vi "挥发酚数据插入.vi"(0 "data":T1={"时间"=timestamp(0 s since 1904-01-01), "测量模式"="水样测试", "数据类型"="N", "检测值"=0.0, "单位"="mg/L", "数据标识"="N", "X0"=0.0, "标样参考值"=0.0, "跨度值"=0.0, "因子编码"="", "X^2"=0.0, "X"=0.0, "B 2"=0.0, "测量量程"=0.0, "测量检出限"=0.0, "测量精度"=0.0, "测量间隔"=0.0, "消解温度"=0.0, "消解时长"=0.0, "三项式系数"=0.0, "二次多项式系数"=0.0, "曲线斜率"=0.0, "曲线截距"=0.0, "线性相关系数"=0.0, "空白校准时间"=timestamp(0 s since 1904-01-01), "标样校准时间"=timestamp(0 s since 1904-01-01), "测量信号值"=0.0, "稀释倍数"=0.0, "量程系数"=0.0, "LastTime"=timestamp(0 s since 1904-01-01), "量程标识"=""}, 3 "错误输入（无错误）":errorcluster) -> (10 "错误输出":errorcluster)   [LabVIEW 2016]
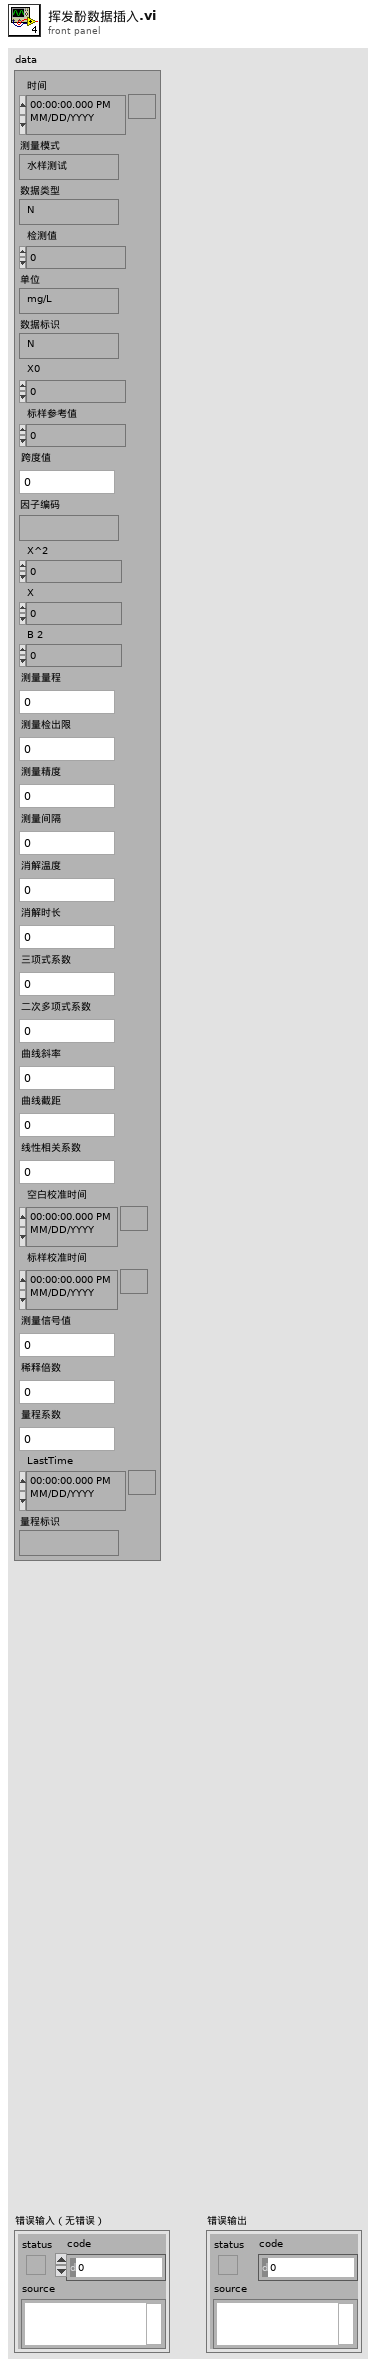
[diagram p1: front panel]
types:
  T1 = cluster{"时间":timestamp, "测量模式":string, "数据类型":string, "检测值":sgl, "单位":string, "数据标识":string, "X0":sgl, "标样参考值":sgl, "跨度值":sgl, "因子编码":string, "X^2":sgl, "X":sgl, "B 2":sgl, "测量量程":sgl, "测量检出限":sgl, "测量精度":sgl, "测量间隔":sgl, "消解温度":sgl, "消解时长":sgl, "三项式系数":sgl, "二次多项式系数":sgl, "曲线斜率":sgl, "曲线截距":sgl, "线性相关系数":sgl, "空白校准时间":timestamp, "标样校准时间":timestamp, "测量信号值":sgl, "稀释倍数":sgl, "量程系数":sgl, "LastTime":timestamp, "量程标识":string}
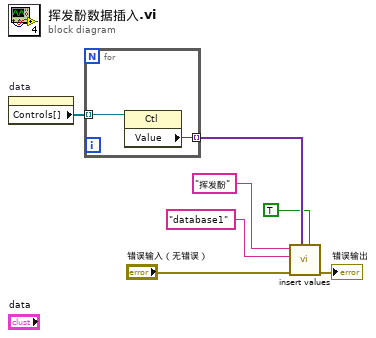
[diagram p0: block diagram]
diagram:
  n1 = property on="data" class="Clust (严格)"() -> ("Controls[]"=w7:refnum<vi>[])  [unwired: 2 in, 2 out]
  n2 = for {
    tunnel: w7 -> [w9] mode=indexing
    tunnel: [w8] -> w6 mode=indexing
    n3 = property class="Ctl"(reference=w9) -> ("Value"=w8:variant)  [unwired: 1 in, 2 out]
  }
  n4 = call "insert values.vi"("是否创建唯一键"=TRUE, "data"=w6, "错误输入（无错误）"="错误输入（无错误）", "database"="database1", "Tabe Name"="挥发酚") -> ("错误输出"=→"错误输出":errorcluster)  [unwired: 6 in]
